vi "main_ctrl.vi"(8 "error in":errorcluster) -> (0 "error out":errorcluster caption="Error")   [LabVIEW 2013]
uses:
  <vilib>/Rock Robotics/WPI/DriverStation/WPI_DriverStationRobotMode2.ctl
  typedefs/fg_typedef.ctl
  typedefs/subStates.ctl
  typedefs/Loop Datatypes/Loop 1 Datatype.ctl
  typedefs/vision enable.ctl
  typedefs/singleUseSubstate.ctl
  <vilib>/Rock Robotics/WPI/Solenoid/WPI_SolenoidValue.ctl
  <vilib>/Rock Robotics/WPI/Compressor/WPI_CompressorGetSetRefNum.vi
  <vilib>/Rock Robotics/WPI/RobotDrive/WPI_RobotDriveGetSetRefNum.vi
  <vilib>/Rock Robotics/WPI/RobotDrive/WPI_RobotDriveArcadeDrive_Standard(NoSaturation).vi
  <vilib>/Rock Robotics/WPI/Solenoid/WPI_SolenoidSetEnum.vi
  typedefs/vision data.ctl
panel:
  out "Robot Mode":T1
  out "Vision SPI":u32
  out "Vision IPS":dbl
  out "Main IPS":dbl
  out "Main SPI":u32
  # "MAIN CONTROL"
  # "holds robot control code - dual parallel state machine"
  # "SPI: milliseconds per iteration\nIPS: iterations per second"
  # "need to incorporate cancel commands"
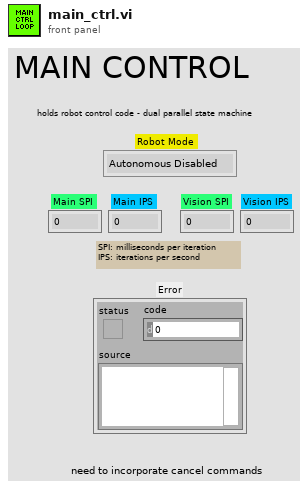
[diagram p1: front panel]
types:
  T1 = typedef "WPI_DriverStationRobotMode2.ctl" = enum16{"Autonomous Disabled", "Autonomous Enabled", "Teleop Disabled", "Teleop Enabled", "Timeout", "Finish", "Test Disabled", "Test Enabled"}
  T2 = typedef "vision data.ctl" = cluster{"x":dbl, "y":dbl, "area":dbl, "width":dbl, "height":dbl, "Hot Goal Present?":bool, "distance":dbl}
  T3 = typedef "vision enable.ctl" = enum16{"Enable", "Disable", "Stop"}
  T4 = typedef "fg_typedef.ctl" = enum16{"Get", "Set"}
  T5 = typedef "WPI_CameraDevRef.ctl" = cluster{"Camera Address":string, "CameraStatus":errorcluster, "Acquire Image Notifier":refnum<notifier>}
  T6 = typedef "IMAQ Image.ctl" = refnum<image>
  T7 = cluster{"Vision mSPI":u32, "Main mSPI":u32, "Dash mSPI":u32}
  T8 = typedef "WPI_RobotDriveDevRef.ctl" = cluster{"DevStatus":errorcluster, "Motors[]":T9[], "Square Inputs":bool, "Max Output":dbl, "Isochronous":bool}
  T9 = typedef "WPI_MotorControlDeviceRef.ctl" = cluster{"DeviceStatus":errorcluster, "Type":enum16{"PWM", "CAN"}, "PWM":cluster{"Digital Module":T10, "PWM Channel":T11, "DeadBand":T12}, "CAN":cluster{"Device Number":u8, "Control Mode":T13, "Semaphore":T14, "Max Vout":dbl}, "Invert":bool, "TransformRef":T15, "InvTransformRef":T15}
  T10 = typedef "FPGA_TypedefDigitalModule.ctl" = enum16{"Digital Module 1", "Digital Module 2"}
  T11 = typedef "FPGA_DIOPWMChannel.ctl" = enum8{"PWM 1", "PWM 2", "PWM 3", "PWM 4", "PWM 5", "PWM 6", "PWM 7", "PWM 8", "PWM 9", "PWM 10", "Invalid"}
  T12 = typedef "WPI_PWMDeadband.ctl" = cluster{"Name":string, "maxPositivePwm":i32, "minPositivePwm":i32, "centerPwm":i32, "maxNegativePwm":i32, "minNegativePwm":i32, "angularRange":u16}
  T13 = typedef "WPI_CANJaguar_ControlMode.ctl" = enum8{"Percent VBus", "Current", "Speed", "Position", "Voltage"}
  T14 = typedef "Semaphore RefNum" = refnum<k1>
  T15 = typedef "WPI_PWMTransform_ConPane.ctl" = refnum<vi>
  T16 = typedef "WPI_DigitalInputDevRef.ctl" = cluster{"DevStatus":errorcluster, "DIO Channel":T17, "Digital Module":T10}
  T17 = typedef "FPGA_DIOChannel.ctl" = enum8{"DIO 1", "DIO 2", "DIO 3", "DIO 4", "DIO 5", "DIO 6", "DIO 7", "DIO 8", "DIO 9", "DIO 10", "DIO 11", "DIO 12", "DIO 13", "DIO 14", "Invalid"}
  T18 = typedef "WPI_SolenoidDevRef.ctl" = cluster{"DevStatus":errorcluster, "Solenoid Module":T19, "Forward Solenoid Channel":T20, "Reverse Solenoid Channel":T20}
  T19 = typedef "FPGA_TypedefSolenoidModule.ctl" = enum16{"Solenoid Module 1", "Solenoid Module 2"}
  T20 = typedef "WPI_SolenoidChannel.ctl" = enum8{"Solenoid 1", "Solenoid 2", "Solenoid 3", "Solenoid 4", "Solenoid 5", "Solenoid 6", "Solenoid 7", "Solenoid 8", "Invalid"}
  T21 = typedef "WPI_CompressorDevRef.ctl" = cluster{"DevStatus":errorcluster, "DigitalInputDevRef":T16, "RelayDevRef":T22}
  T22 = typedef "WPI_RelayDevRef.ctl" = cluster{"DevStatus":errorcluster, "Relay Channel":T23, "Digital Module":T10, "Relay Direction":T24}
  T23 = typedef "FPGA_DIORelayChannel.ctl" = enum8{"Relay 1", "Relay 2", "Relay 3", "Relay 4", "Relay 5", "Relay 6", "Relay 7", "Relay 8", "Invalid"}
  T24 = typedef "WPI_RelayDirection.ctl" = enum16{"Both directions", "Forward only", "Reverse only"}
  T25 = typedef "Loop 1 Datatype.ctl" = cluster{"State":T26, "Waiting Loop":i32, "State to Wait For":i32, "Loop ID":i32, "Exit Value":i32}
  T26 = typedef "subStates.ctl" = enum16{"null", "wait", "driver control", "auto", "manual override", "hold position", "rotate", "pickup", "pass", "load", "goto shoot", "shoot", "cancel", "end"}
  T27 = typedef "WPI_SolenoidValue.ctl" = enum16{"Off", "On", "Forward", "Reverse"}
  T28 = typedef "singleUseSubstate.ctl" = enum16{"null", "wait", "shift high", "shift low", "extend shooter", "retract shooter", "close latch", "open latch"}
  T29 = typedef "WPI_DriverStationDerivedRobotMode.ctl" = enum16{"Init", "Execute", "Stop"}
  T30 = typedef "Loop 2 Datatype.ctl" = cluster{"State":T26, "Waiting Loop":i32, "State to Wait For":i32, "Loop ID":i32, "Exit Value":i32, "Joystick Y":dbl, "Tune Speed":dbl}
  T31 = typedef "Loop 3 Datatype.ctl" = cluster{"State":T26, "Waiting Loop":i32, "State to Wait For":i32, "Loop ID":i32, "Exit Value":i32, "Joystick Y":dbl, "Joystick Z":dbl}
  T32 = typedef "Loop 0 Datatype.ctl" = cluster{"State":T26, "Waiting Loop":i32, "State to Wait For":i32, "Loop ID":i32, "Exit Value":i32, "X Axis":dbl, "Y Axis":dbl, "Z Axis":dbl}
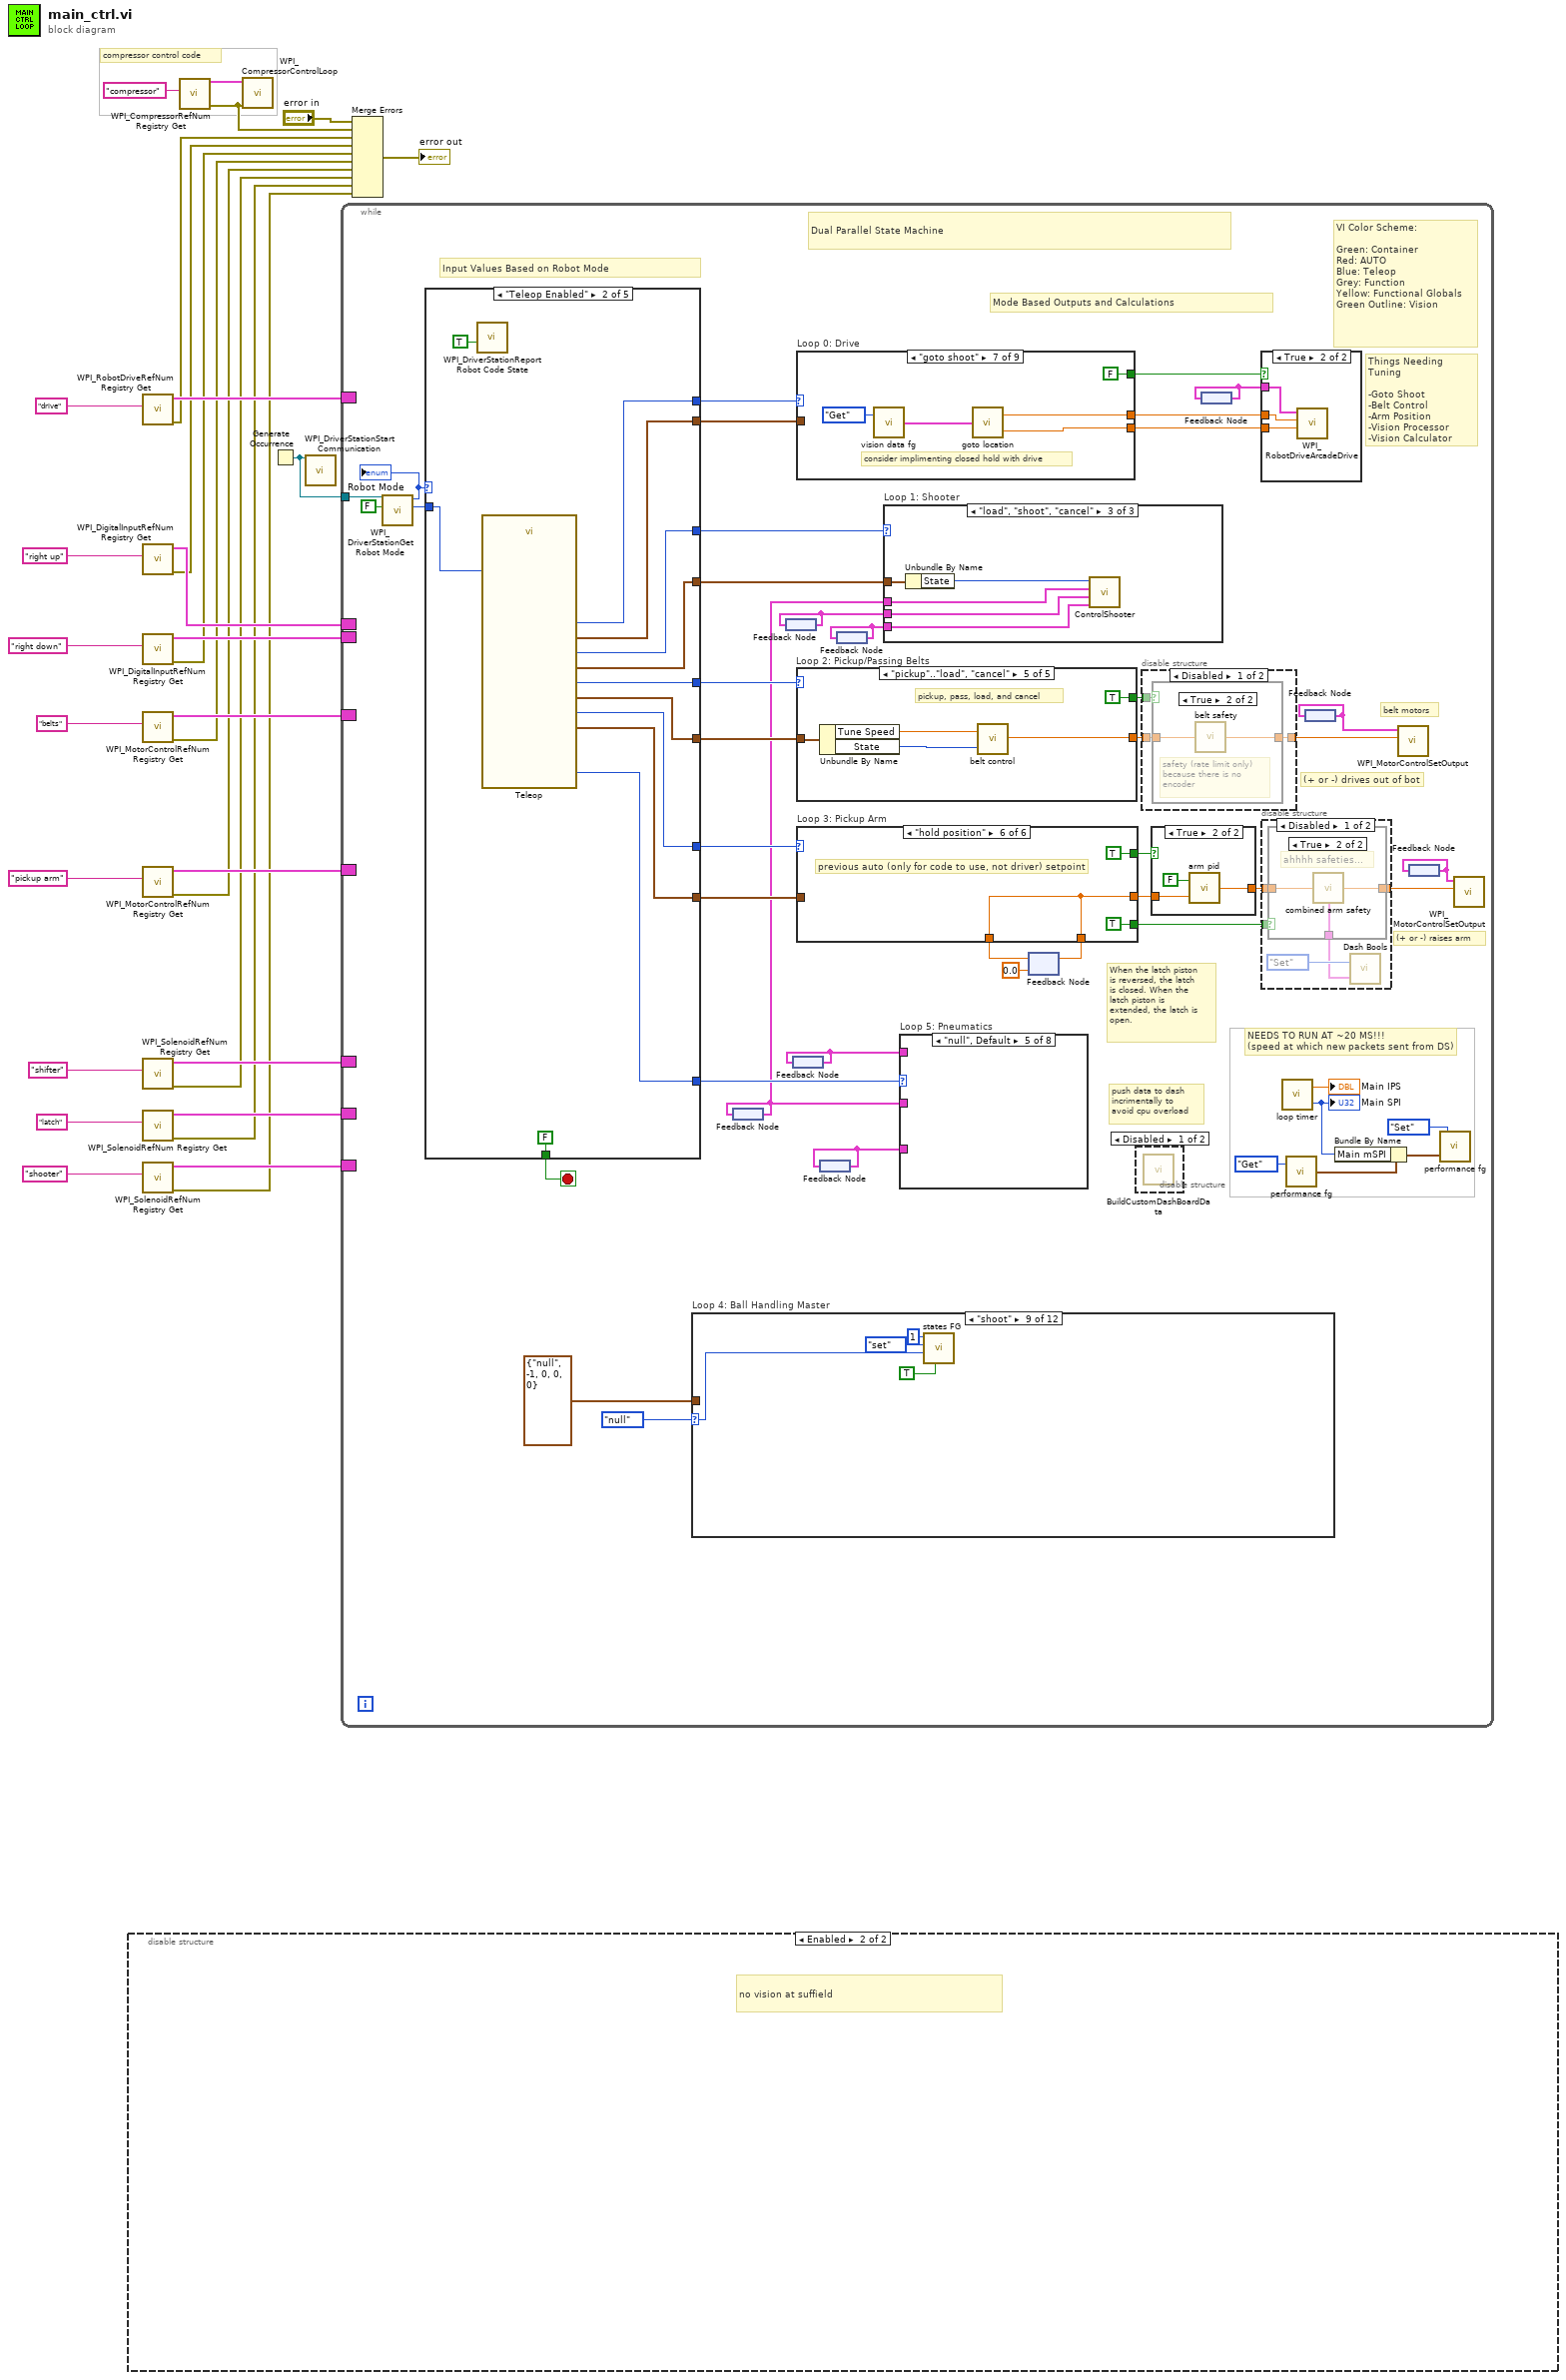
[diagram p0: block diagram]
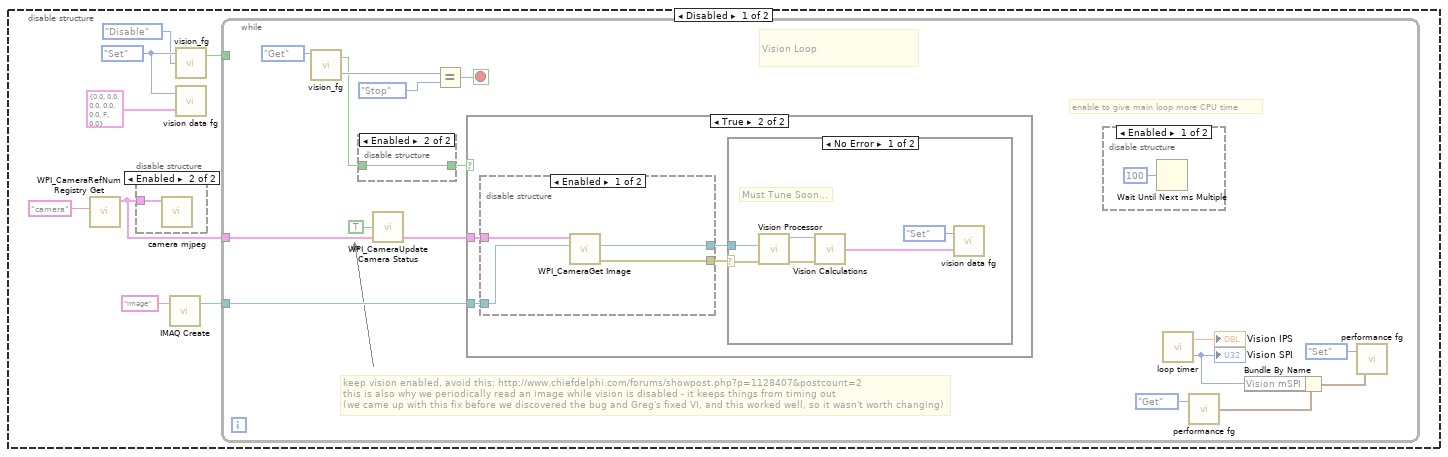
[diagram p2: hidden frame]
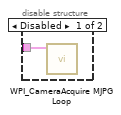
[diagram p3: hidden frame]
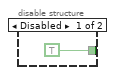
[diagram p4: hidden frame]
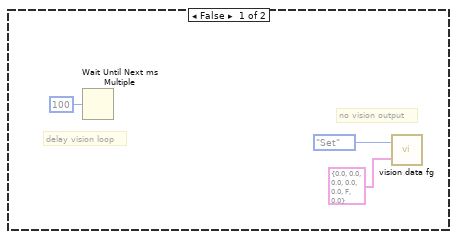
[diagram p6: hidden frame]
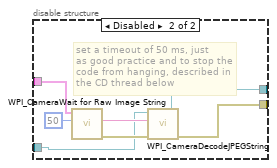
[diagram p8: hidden frame]
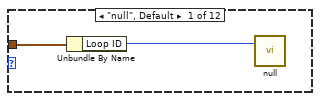
[diagram p9: hidden frame]
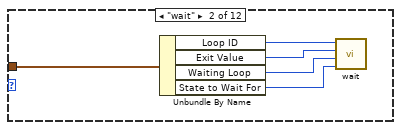
[diagram p10: hidden frame]
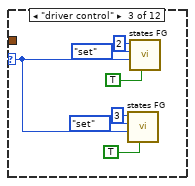
[diagram p11: hidden frame]
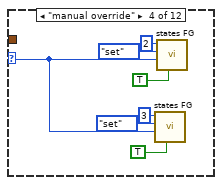
[diagram p12: hidden frame]
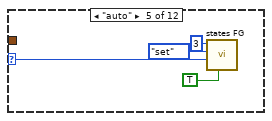
[diagram p13: hidden frame]
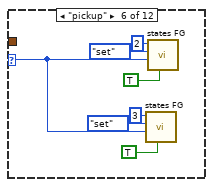
[diagram p14: hidden frame]
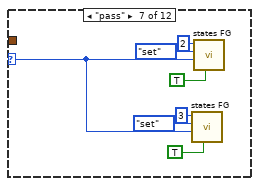
[diagram p15: hidden frame]
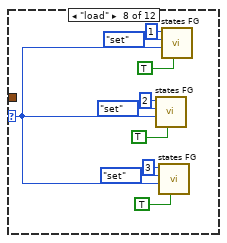
[diagram p16: hidden frame]
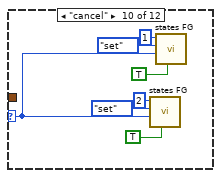
[diagram p17: hidden frame]
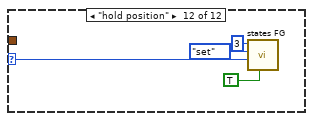
[diagram p19: hidden frame]
diagram:
  # "compressor control code"
  n1 = disable-structure shown="Enabled" {
    frame Disabled {
      w36 = fg_typedef."Set" ("Enum")
      n2 = call <vilib>:"WPI_CameraRefNum Registry Get.vi"("refnum name"="camera") -> ("CameraDevRef"=w33:T5)  [unwired: 9 in, 1 out]
      n3 = disable-structure shown="Enabled" {
        disable-tunnel: w33 -> [w39 w40]
        frame Disabled {
          n4 = call <vilib>:"WPI_CameraAcquire MJPG Loop.vi"("CameraDevRef"=w39) -> ()  [unwired: 11 in]
        }
        frame Enabled {
          n5 = call "camera mjpeg.vi"("CameraDevRef"=w40) -> ()  [unwired: 11 in]
        }
      }
      n6 = call "IMAQ Create"("Image Name"="image") -> ("New Image"=w38:T6)  [unwired: 4 in, 1 out]
      n7 = call "vision_fg.vi"("Action"=vision_enable."Disable", "Menu"=w36) -> ("Enabled?"=w37:bool)  [unwired: 1 in, 1 out]
      n8 = call "vision data fg.vi"("Input"=T2 {"x"=0.0, "y"=0.0, "area"=0.0, "width"=0.0, "height"=0.0, "Hot Goal Present?"=FALSE, "distance"=0.0} ("Cluster"), "Menu"=w36) -> ()  [unwired: 1 out]
      n9 = while {
        tunnel: w38 -> [w55]
        tunnel: w33 -> [w54]
        tunnel: w37 -> [_]
        stop <- w56 stop-if-true
        # "keep vision enabled, avoid this: http://www.chiefdelphi.com/forums/showpost.php?p=1128407&postcount=2\nthis is also why we periodically read an image while vision is disabled - it keeps things from timing out\n(we came up with this fix before we discovered the bug and Greg's fixed VI, and this worked well, so it wasn't worth changing)"
        # "enable to give main loop more CPU time"
        # "Vision Loop"
        n10 = call "vision_fg.vi"("Menu"=fg_typedef."Get" ("Enum")) -> ("State Out"=w50:T3, "Enabled?"=w41:bool)  [unwired: 2 in]
        n11 = disable-structure shown="Enabled" {
          disable-tunnel: [TRUE w58] -> w42
          disable-tunnel: w41 -> [_ w58]
          frame Disabled {
          }
          frame Enabled {
          }
        }
        n12 = call <vilib>:"WPI_CameraUpdate Camera Status.vi"("CameraDevRef In"=w54, "Enable Vision"=TRUE) -> ("CameraDevRef Out"=w53:T5)  [unwired: 3 in]
        n13 = Equal?(x=w50, y=vision_enable."Stop") -> (x = y?=w56:bool)
        n14 = case shown="True" w42 {
          tunnel: w55 -> [_ w66]
          tunnel: w53 -> [_ w65]
          frame False {
            # "no vision output"
            # "delay vision loop"
            n15 = Wait Until Next ms Multiple(millisecond multiple=u32 100) -> ()  [unwired: 1 out]
            n16 = call "vision data fg.vi"("Input"=T2 {"x"=0.0, "y"=0.0, "area"=0.0, "width"=0.0, "height"=0.0, "Hot Goal Present?"=FALSE, "distance"=0.0} ("Cluster"), "Menu"=fg_typedef."Set" ("Enum")) -> ()  [unwired: 1 out]
          }
          frame True {
            n17 = disable-structure shown="Enabled" {
              disable-tunnel: w66 -> [w75 w79]
              disable-tunnel: w65 -> [w76 w81]
              disable-tunnel: [w74 w78] -> w64
              disable-tunnel: [w73 w77] -> w63
              frame Enabled {
                n18 = call <vilib>:"WPI_CameraGet Image.vi"("Image"=w75, "CameraDevRef"=w76) -> ("error out"=w73:errorcluster, "Image Out"=w74:T6)  [unwired: 7 in, 1 out]
              }
              frame Disabled {
                # "set a timeout of 50 ms, just\nas good practice and to stop the \ncode from hanging, described in \nthe CD thread below"
                n19 = call <vilib>:"WPI_CameraWait for Raw Image String.vi"("Timeout in ms (-1)"=50, "CameraDevRef"=w81) -> ("error out"=w83:errorcluster, "String"=w82:string)  [unwired: 3 in, 5 out]
                n20 = call <vilib>:"WPI_CameraDecodeJPEGString.vi"("error in"=w83, "Compressed Image"=w82, "Image In"=w79) -> ("error out"=w77:errorcluster, "Image Out"=w78:T6)  [unwired: 3 out]
              }
            }
            n21 = case shown="No Error" w63 {
              selector: w63 -> [w71 _]
              tunnel: w64 -> [w70 _]
              frame No Error {
                # "Must Tune Soon..."
                n22 = call "Vision Processor.vi"("error in"=w71, "Image In"=w70) -> ("error out"=w68:errorcluster, "Image Out"=w69:T6)  [unwired: 5 in]
                n23 = call "Vision Calculations.vi"("Image In"=w69, "error in"=w68) -> ("Vision Data"=w67:T2)  [unwired: 3 in]
                n24 = call "vision data fg.vi"("Input"=w67, "Menu"=fg_typedef."Set" ("Enum")) -> ()  [unwired: 1 out]
              }
              frame Error {
              }
            }
          }
        }
        n25 = disable-structure shown="Enabled" {
          frame Enabled {
            n26 = Wait Until Next ms Multiple(millisecond multiple=u32 100) -> ()  [unwired: 1 out]
          }
          frame Disabled {
          }
        }
        n27 = call "loop timer.vi"() -> ("IPS"=→"Vision IPS":dbl, "SPI"=w48:u32)  [unwired: 1 in]
        "Vision SPI" <- w48
        n28 = call "performance fg.vi"("Menu"=fg_typedef."Get") -> ("Output"=w46:T7)  [unwired: 1 in]
        n29 = Bundle By Name(cluster=w46, "Vision mSPI"=w48) -> (w45:T7)
        n30 = call "performance fg.vi"("Input"=w45, "Menu"=fg_typedef."Set") -> ()  [unwired: 1 out]
      }
    }
    frame Enabled {
      # "no vision at suffield"
    }
  }
  n31 = call <vilib>:"WPI_RobotDriveRefNum Registry Get.vi"("refnum name"="drive") -> ("error out"=w10:errorcluster, "RobotDriveDevRef"=w27:T8)  [unwired: 9 in]
  n32 = call <vilib>:"WPI_DigitalInputRefNum Registry Get.vi"("refnum name"="right up") -> ("error out"=w9:errorcluster, "DigitalInputDevRef"=w12:T16)  [unwired: 9 in]
  n33 = call <vilib>:"WPI_DigitalInputRefNum Registry Get.vi"("refnum name"="right down") -> ("error out"=w8:errorcluster, "DigitalInputDevRef"=w11:T16)  [unwired: 9 in]
  n34 = call <vilib>:"WPI_MotorControlRefNum Registry Get.vi"("refnum name"="belts") -> ("error out"=w7:errorcluster, "MotorControlDevRef"=w18:T9)  [unwired: 9 in]
  n35 = call <vilib>:"WPI_MotorControlRefNum Registry Get.vi"("refnum name"="pickup arm") -> ("error out"=w6:errorcluster, "MotorControlDevRef"=w15:T9)  [unwired: 9 in]
  n36 = call <vilib>:"WPI_SolenoidRefNum Registry Get.vi"("refnum name"="shifter") -> ("error out"=w5:errorcluster, "SolenoidDevRef"=w25:T18)  [unwired: 9 in]
  n37 = call <vilib>:"WPI_SolenoidRefNum Registry Get.vi"("refnum name"="latch") -> ("error out"=w4:errorcluster, "SolenoidDevRef"=w19:T18)  [unwired: 9 in]
  n38 = call <vilib>:"WPI_SolenoidRefNum Registry Get.vi"("refnum name"="shooter") -> ("error out"=w3:errorcluster, "SolenoidDevRef"=w21:T18)  [unwired: 9 in]
  n39 = call <vilib>:"WPI_CompressorRefNum Registry Get.vi"("refnum name"="compressor") -> ("error out"=w1:errorcluster, "CompressorDevRef"=w26:T21)  [unwired: 9 in]
  n40 = call <vilib>:"WPI_CompressorControlLoop.vi"("error in (no error)"=w1, "CompressorDevRef"=w26) -> ()  [unwired: 10 in]
  n41 = Generate Occurrence() -> (w23:refnum<k4>)
  n42 = call <vilib>:"WPI_DriverStationStart Communication.vi"("occurrence"=w23) -> ()  [unwired: 11 in]
  n43 = while {
    tunnel: w23 -> [w105]
    border: w27 -> [_]
    border: w25 -> [_]
    border: w21 -> [_]
    border: w19 -> [_]
    border: w18 -> [_]
    border: w15 -> [_]
    border: w12 -> [_]
    border: w11 -> [_]
    stop <- w124 stop-if-true
    # "When the latch piston\nis reversed, the latch\nis closed. When the\nlatch piston is\nextended, the latch is\nopen."
    # "push data to dash \nincrimentally to\navoid cpu overload"
    # "Things Needing Tuning\n\n-Goto Shoot\n-Belt Control\n-Arm Position\n-Vision Processor\n-Vision Calculator"
    # "(+ or -) raises arm"
    # "(+ or -) drives out of bot"
    # "belt motors"
    # "VI Color Scheme:\n\nGreen: Container\nRed: AUTO\nBlue: Teleop\nGrey: Function\nYellow: Functional Globals\nGreen Outline: Vision"
    # "Input Values Based on Robot Mode"
    # "Mode Based Outputs and Calculations"
    # "NEEDS TO RUN AT ~20 MS!!!\n(speed at which new packets sent from DS)"
    # "Dual Parallel State Machine"
    n44 = call <vilib>:"WPI_DriverStationGet Robot Mode.vi"("Finish"=FALSE, "DS Occurrence"=w105) -> ("Call Context"=w104:T29, "Robot Mode"=w103:T1)  [unwired: 8 out]
    "Robot Mode" <- w103
    n45 = case shown="\"Teleop Enabled\"" w103 {
      tunnel: [w378 w393 w395 w401 w407] -> w107
      tunnel: w104 -> [w371 w389 _ _ _]
      tunnel: [w376 w392 w395 w401 w407] -> w126
      tunnel: [w372 w390 singleUseSubstate."null" ("SubState 5") singleUseSubstate."null" ("SubState 5") singleUseSubstate."null" ("SubState 5")] -> w125
      tunnel: [FALSE FALSE FALSE FALSE TRUE] -> w124
      tunnel: [w380 w388 w395 w401 w407] -> w117
      tunnel: [w379 w387 _ _ _] -> w118
      tunnel: [w377 w386 _ _ _] -> w116
      tunnel: [w375 w385 _ _ _] -> w115
      tunnel: [w373 w384 _ _ _] -> w113
      tunnel: [w374 w383 w395 w401 w407] -> w112
      frame "Autonomous Enabled" {
        n46 = call <vilib>:"WPI_DriverStationReport Robot Code State.vi"("Autonomous"=TRUE) -> ()  [unwired: 10 in, 1 out]
        n47 = call "Autonomous.vi"("Call Context"=w371) -> ("SubState 2"=w376:T26, "Loop 2 Data"=w375:T30, "SubState 1"=w378:T26, "Loop 1 Data"=w377:T25, "Loop 3 Data"=w373:T31, "SubState 0"=w380:T26, "SubState 3"=w374:T26, "Loop 0 Data"=w379:T32, "SubState 5"=w372:T28)  [unwired: 2 out]
      }
      frame "Teleop Enabled" {
        n48 = call <vilib>:"WPI_DriverStationReport Robot Code State.vi"("TeleOp"=TRUE) -> ()  [unwired: 10 in, 1 out]
        n49 = call "Teleop.vi"("Call Context"=w389) -> ("SubState 3"=w383:T26, "SubState 5"=w390:T28, "Loop 3 Data"=w384:T31, "SubState 0"=w388:T26, "Loop 1 Data"=w386:T25, "Loop 0 Data"=w387:T32, "SubState 1"=w393:T26, "Loop 2 Data"=w385:T30, "SubState 2"=w392:T26)  [unwired: 8 in, 2 out]
      }
      frame "Autonomous Disabled", "Teleop Disabled", "Timeout" {
        w395 = subStates."null" ("SubState 0")
        # "set all loops to null"
        # "make sure to disable vision\nwe don't need it here"
        # "robot disabled, timeout"
        n50 = call <vilib>:"WPI_DriverStationReport Robot Code State.vi"("Disabled"=TRUE) -> ()  [unwired: 10 in, 1 out]
        n51 = call "vision_fg.vi"("Action"=vision_enable."Disable", "Menu"=fg_typedef."Set") -> ()  [unwired: 1 in, 2 out]
      }
      frame "Test Disabled", "Test Enabled" {
        w401 = subStates."null" ("SubState 0")
        # "set all loops to null"
        # "make sure to disable vision\nwe don't need it here"
        # "test, unused"
        n52 = call <vilib>:"WPI_DriverStationReport Robot Code State.vi"("Test"=TRUE) -> ()  [unwired: 10 in, 1 out]
        n53 = call "vision_fg.vi"("Action"=vision_enable."Disable", "Menu"=fg_typedef."Set") -> ()  [unwired: 1 in, 2 out]
      }
      frame "Finish" {
        w407 = subStates."end"  # Stop All Loops
        # "stop the while loop"
        # "stop DS comms"
        # "stop vision loop"
        n54 = call <vilib>:"WPI_DriverStationStop Communication.vi"("StopCommunication"=TRUE) -> ()  [unwired: 10 in, 1 out]
        n55 = call "vision_fg.vi"("Action"=vision_enable."Stop", "Menu"=fg_typedef."Set") -> ()  [unwired: 1 in, 2 out]
      }
    }
    n56 = case "Loop 4: Ball Handling Master" shown="\"shoot\"" subStates."null" ("Stop All Loops") {
      selector: subStates."null" ("Stop All Loops") -> [_ _ w135 w142 w149 w153 w160 w167 w177 w181 _ w188]
      tunnel: T25 {"State"=enum."null", "Waiting Loop"=-1, "State to Wait For"=0, "Loop ID"=0, "Exit Value"=0} ("input cluster") -> [w129 w130 _ _ _ _ _ _ _ _ _ _]
      frame "null", Default {
        n57 = Unbundle By Name(w129) -> ("Loop ID"=w128:i32)
        n58 = call "null.vi"("This Loop ID"=w128) -> ()  [unwired: 2 in]
      }
      frame "wait" {
        n59 = Unbundle By Name(w130) -> ("Loop ID"=w134:i32, "Exit Value"=w133:i32, "Waiting Loop"=w132:i32, "State to Wait For"=w131:i32)
        n60 = call "wait.vi"("State to wait for"=w131, "Waiting Loop ID"=w132, "time (ms)"=w133, "Current Loop ID"=w134) -> ()  [unwired: 1 out]
      }
      frame "driver control" {
        n61 = call "states FG.vi"("exit in"=TRUE, "subState in"=w135, "menu (get)"=enum16{"set", "get"}."set", "Loop ID"=3) -> ()  [unwired: 4 in, 4 out]
        n62 = call "states FG.vi"("exit in"=TRUE, "subState in"=w135, "menu (get)"=enum16{"set", "get"}."set", "Loop ID"=2) -> ()  [unwired: 4 in, 4 out]
      }
      frame "manual override" {
        n63 = call "states FG.vi"("exit in"=TRUE, "subState in"=w142, "menu (get)"=enum16{"set", "get"}."set", "Loop ID"=3) -> ()  [unwired: 4 in, 4 out]
        n64 = call "states FG.vi"("exit in"=TRUE, "subState in"=w142, "menu (get)"=enum16{"set", "get"}."set", "Loop ID"=2) -> ()  [unwired: 4 in, 4 out]
      }
      frame "auto" {
        n65 = call "states FG.vi"("exit in"=TRUE, "subState in"=w149, "menu (get)"=enum16{"set", "get"}."set", "Loop ID"=3) -> ()  [unwired: 4 in, 4 out]
      }
      frame "pickup" {
        n66 = call "states FG.vi"("exit in"=TRUE, "subState in"=w153, "menu (get)"=enum16{"set", "get"}."set", "Loop ID"=3) -> ()  [unwired: 4 in, 4 out]
        n67 = call "states FG.vi"("exit in"=TRUE, "subState in"=w153, "menu (get)"=enum16{"set", "get"}."set", "Loop ID"=2) -> ()  [unwired: 4 in, 4 out]
      }
      frame "pass" {
        n68 = call "states FG.vi"("exit in"=TRUE, "subState in"=w160, "menu (get)"=enum16{"set", "get"}."set", "Loop ID"=3) -> ()  [unwired: 4 in, 4 out]
        n69 = call "states FG.vi"("exit in"=TRUE, "subState in"=w160, "menu (get)"=enum16{"set", "get"}."set", "Loop ID"=2) -> ()  [unwired: 4 in, 4 out]
      }
      frame "load" {
        n70 = call "states FG.vi"("exit in"=TRUE, "subState in"=w167, "menu (get)"=enum16{"set", "get"}."set", "Loop ID"=2) -> ()  [unwired: 4 in, 4 out]
        n71 = call "states FG.vi"("exit in"=TRUE, "subState in"=w167, "menu (get)"=enum16{"set", "get"}."set", "Loop ID"=3) -> ()  [unwired: 4 in, 4 out]
        n72 = call "states FG.vi"("exit in"=TRUE, "subState in"=w167, "menu (get)"=enum16{"set", "get"}."set", "Loop ID"=1) -> ()  [unwired: 4 in, 4 out]
      }
      frame "shoot" {
        n73 = call "states FG.vi"("exit in"=TRUE, "subState in"=w177, "menu (get)"=enum16{"set", "get"}."set", "Loop ID"=1) -> ()  [unwired: 4 in, 4 out]
      }
      frame "cancel" {
        n74 = call "states FG.vi"("exit in"=TRUE, "subState in"=w181, "menu (get)"=enum16{"set", "get"}."set", "Loop ID"=2) -> ()  [unwired: 4 in, 4 out]
        n75 = call "states FG.vi"("exit in"=TRUE, "subState in"=w181, "menu (get)"=enum16{"set", "get"}."set", "Loop ID"=1) -> ()  [unwired: 4 in, 4 out]
      }
      frame "end" {
      }
      frame "hold position" {
        n76 = call "states FG.vi"("exit in"=TRUE, "subState in"=w188, "menu (get)"=enum16{"set", "get"}."set", "Loop ID"=3) -> ()  [unwired: 4 in, 4 out]
      }
    }
    n77 = feedback #1() -> (w86:T18)
    n78 = feedback-in #1(w86) -> ()
    n79 = feedback #2() -> (w88:T16)
    n80 = feedback-in #2(w88) -> ()
    n81 = feedback #3() -> (w114:T18)
    n82 = feedback-in #3(w114) -> ()
    n83 = case "Loop 0: Drive" shown="\"goto shoot\"" w117 {
      tunnel: w118 -> [w222 w226 w238 w245 w262 w269 _ _ w285]
      tunnel: [w220 w224 w236 w247 w259 w271 w274 w279 w281] -> w110
      tunnel: [w220 w224 w235 w246 w258 w270 w273 w279 w280] -> w109
      tunnel: [FALSE FALSE TRUE FALSE FALSE FALSE FALSE FALSE FALSE] -> w111
      frame "null", Default {
        w220 = 0.0 ("X Axis")
        n84 = Unbundle By Name(w222) -> ("Loop ID"=w223:i32)
        n85 = call "null.vi"("This Loop ID"=w223) -> ()  [unwired: 2 in]
      }
      frame "wait" {
        w224 = 0.0 ("X Axis")
        n86 = Unbundle By Name(w226) -> ("Loop ID"=w230:i32, "Exit Value"=w229:i32, "Waiting Loop"=w228:i32, "State to Wait For"=w227:i32)
        n87 = call "wait.vi"("State to wait for"=w227, "Waiting Loop ID"=w228, "time (ms)"=w229, "Current Loop ID"=w230) -> ()  [unwired: 1 out]
      }
      frame "driver control" {
        # "filter joysticks"
        n88 = Unbundle By Name(w238) -> ("X Axis"=w231:dbl, "Y Axis"=w234:dbl)
        n89 = call "Joystick Error Filter.vi"("Axis"=w231) -> ("Filtered Axis"=w232:dbl)
        n90 = call "Joystick Error Filter.vi"("Axis"=w234) -> ("Filtered Axis"=w233:dbl)
        n91 = disable-structure shown="Enabled" {
          disable-tunnel: w232 -> [w242 w244]
          disable-tunnel: w233 -> [w241 w243]
          disable-tunnel: [w240 w244] -> w236
          disable-tunnel: [w239 w243] -> w235
          frame Disabled {
            n92 = call "calc arcade drive pwm.vi"("Y axis value"=w241, "X axis value"=w242) -> ("Right Speed"=w239:dbl, "Left Speed"=w240:dbl)  [unwired: 1 in, 1 out]
          }
          frame Enabled {
          }
        }
      }
      frame "auto" {
        n93 = disable-structure shown="Enabled" {
          disable-tunnel: [w256 _] -> w247
          disable-tunnel: [w255 _] -> w246
          disable-tunnel: w245 -> [w251 _]
          frame Disabled {
            n94 = Unbundle By Name(w251) -> ("Z Axis"=w249:dbl)
            n95 = call "Vision Tracking X.vi"("Tweak"=w249) -> ("right speed"=w250:dbl, "left speed"=w253:dbl)
            n96 = call "closed drive.vi"("Acrade Drive?"=FALSE, "Y axis value (Left)"=w253, "X axis value (Right)"=w250, "Threshold (.4)"=0.0 ("Threshold")) -> ("right"=w255:dbl, "left"=w256:dbl)
          }
          frame Enabled {
            # "rotates toward target"
            # "not in use this year"
          }
        }
      }
      frame "hold position" {
        n97 = Unbundle By Name(w262) -> ("X Axis"=w261:dbl, "Y Axis"=w260:dbl)
        n98 = call "closed drive.vi"("Acrade Drive?"=TRUE, "Y axis value (Left)"=w260, "X axis value (Right)"=w261) -> ("right"=w258:dbl, "left"=w259:dbl)  [unwired: 1 in]
      }
      frame "rotate" {
        # "use these to carry actual information because this is\nfor autonomous only so there will not be joystick input"
        n99 = Unbundle By Name(w269) -> ("X Axis"=w268:dbl, "Y Axis"=w267:dbl)
        n100 = call "rotate.vi"("Angle"=w268, "Rate"=w267) -> ("finished?"=w264:bool, "left speed"=w271:dbl, "right speed"=w270:dbl)
        n101 = call "states FG.vi"("exit in"=w264, "menu (get)"=enum16{"set", "get"}."set", "Loop ID"=0) -> ()  [unwired: 5 in, 4 out]
      }
      frame "goto shoot" {
        # "consider implimenting closed hold with drive"
        n102 = call "vision data fg.vi"("Menu"=fg_typedef."Get") -> ("Output"=w275:T2)  [unwired: 1 in]
        n103 = call "goto location.vi"("Image Data"=w275) -> ("left speed"=w274:dbl, "right speed"=w273:dbl)
      }
      frame "end" {
        w279 = 0.0 ("X Axis")
      }
      frame "manual override" {
        n104 = Unbundle By Name(w285) -> ("X Axis"=w284:dbl, "Y Axis"=w283:dbl)
        n105 = expression code="x/2"(w284) -> (w281:dbl)
        n106 = expression code="x/2"(w283) -> (w280:dbl)
      }
    }
    n107 = case "Loop 2: Pickup/Passing Belts" shown="\"pickup\"..\"load\", \"cancel\"" w126 {
      tunnel: w115 -> [w337 w340 w348 w352 w357]
      tunnel: [0.0 ("output") 0.0 ("output") w346 w350 w354] -> w94
      tunnel: [FALSE FALSE TRUE FALSE TRUE] -> w95
      frame "null", Default {
        n108 = Unbundle By Name(w337) -> ("Loop ID"=w336:i32)
        n109 = call "null.vi"("This Loop ID"=w336) -> ()  [unwired: 2 in]
      }
      frame "wait" {
        n110 = Unbundle By Name(w340) -> ("Loop ID"=w344:i32, "Exit Value"=w343:i32, "Waiting Loop"=w342:i32, "State to Wait For"=w341:i32)
        n111 = call "wait.vi"("State to wait for"=w341, "Waiting Loop ID"=w342, "time (ms)"=w343, "Current Loop ID"=w344) -> ()  [unwired: 1 out]
      }
      frame "driver control" {
        n112 = Unbundle By Name(w348) -> ("Joystick Y"=w345:dbl)
        n113 = call "Joystick Error Filter.vi"("Axis"=w345) -> ("Filtered Axis"=w346:dbl)
      }
      frame "manual override" {
        n114 = Unbundle By Name(w352) -> ("Joystick Y"=w351:dbl)
        n115 = expression code="x/2"(w351) -> (w350:dbl)
      }
      frame "pickup".."load", "cancel" {
        # "pickup, pass, load, and cancel"
        n116 = Unbundle By Name(w357) -> ("Tune Speed"=w356:dbl, "State"=w355:T26)
        n117 = call "belt control.vi"("State"=w355, "Joystick Z"=w356) -> ("output"=w354:dbl)
      }
    }
    n118 = feedback #4() -> (w89:T18)
    n119 = feedback-in #4(w89) -> ()
    n120 = feedback #5() -> (w87:T16)
    n121 = feedback-in #5(w87) -> ()
    n122 = case "Loop 1: Shooter" shown="\"load\", \"shoot\", \"cancel\"" w107 {
      tunnel: w116 -> [w358 w360 w369]
      tunnel: w86 -> [_ _ w367]
      tunnel: w88 -> [_ _ w366]
      tunnel: w87 -> [_ _ w365]
      frame "null", Default {
        n123 = Unbundle By Name(w358) -> ("Loop ID"=w359:i32)
        n124 = call "null.vi"("This Loop ID"=w359) -> ()  [unwired: 2 in]
      }
      frame "wait" {
        n125 = Unbundle By Name(w360) -> ("Loop ID"=w364:i32, "Exit Value"=w363:i32, "Waiting Loop"=w362:i32, "State to Wait For"=w361:i32)
        n126 = call "wait.vi"("State to wait for"=w361, "Waiting Loop ID"=w362, "time (ms)"=w363, "Current Loop ID"=w364) -> ()  [unwired: 1 out]
      }
      frame "load", "shoot", "cancel" {
        n127 = Unbundle By Name(w369) -> ("State"=w368:T26)
        n128 = call "ControlShooter.vi"("right down"=w365, "right up"=w366, "latch"=w367, "State"=w368) -> ()  [unwired: 1 in]
      }
    }
    n129 = case "Loop 5: Pneumatics" shown="\"null\", Default" w125 {
      tunnel: w114 -> [_ _ _ _ _ _ w331 w332]
      tunnel: w86 -> [w322 w324 _ _ _ _ _ _]
      tunnel: w89 -> [_ _ w326 w328 _ _ _ _]
      frame "open latch" {
        n130 = call-poly <vilib>:"WPI_SolenoidSet.vi"("Value"=WPI_SolenoidValue."Forward", "SolenoidDevRef"=w322) -> ()  [unwired: 8 in, 2 out]
      }
      frame "close latch" {
        n131 = call-poly <vilib>:"WPI_SolenoidSet.vi"("Value"=WPI_SolenoidValue."Forward", "SolenoidDevRef"=w324) -> ()  [unwired: 8 in, 2 out]
      }
      frame "retract shooter" {
        n132 = call-poly <vilib>:"WPI_SolenoidSet.vi"("Value"=WPI_SolenoidValue."Reverse", "SolenoidDevRef"=w326) -> ()  [unwired: 8 in, 2 out]
      }
      frame "extend shooter" {
        n133 = call-poly <vilib>:"WPI_SolenoidSet.vi"("Value"=WPI_SolenoidValue."Forward", "SolenoidDevRef"=w328) -> ()  [unwired: 8 in, 2 out]
      }
      frame "null", Default {
      }
      frame "wait" {
      }
      frame "shift high" {
        n134 = call-poly <vilib>:"WPI_SolenoidSet.vi"("Value"=WPI_SolenoidValue."Forward", "SolenoidDevRef"=w331) -> ()  [unwired: 8 in, 2 out]
      }
      frame "shift low" {
        n135 = call-poly <vilib>:"WPI_SolenoidSet.vi"("Value"=WPI_SolenoidValue."Reverse", "SolenoidDevRef"=w332) -> ()  [unwired: 8 in, 2 out]
      }
    }
    n136 = feedback #6(0.0 ("setpoint")) -> (w91:dbl)
    n137 = case "Loop 3: Pickup Arm" shown="\"hold position\"" w112 {
      tunnel: w113 -> [w291 w296 w305 w312 w318 _]
      tunnel: [FALSE FALSE FALSE FALSE TRUE TRUE] -> w100
      tunnel: [0.0 ("output") 0.0 ("output") w302 w310 w313 w319] -> w99
      tunnel: [TRUE TRUE TRUE FALSE TRUE TRUE] -> w98
      tunnel: [w286 w292 w301 w307 w313 w319] -> w92
      tunnel: w91 -> [w286 w292 w301 w307 _ w319]
      frame "null", Default {
        n138 = Unbundle By Name(w291) -> ("Loop ID"=w290:i32)
        n139 = call "null.vi"("This Loop ID"=w290) -> ()  [unwired: 2 in]
      }
      frame "wait" {
        n140 = Unbundle By Name(w296) -> ("Loop ID"=w300:i32, "Exit Value"=w299:i32, "Waiting Loop"=w298:i32, "State to Wait For"=w297:i32)
        n141 = call "wait.vi"("State to wait for"=w297, "Waiting Loop ID"=w298, "time (ms)"=w299, "Current Loop ID"=w300) -> ()  [unwired: 1 out]
      }
      frame "driver control" {
        n142 = Unbundle By Name(w305) -> ("Joystick Y"=w303:dbl)
        n143 = call "Joystick Error Filter.vi"("Axis"=w303) -> ("Filtered Axis"=w302:dbl)
      }
      frame "manual override" {
        n144 = Unbundle By Name(w312) -> ("Joystick Y"=w311:dbl)
        n145 = expression code="x/2"(w311) -> (w310:dbl)
      }
      frame "auto", "pickup".."load" {
        # "pickup, pass, auto, and load"
        n146 = Unbundle By Name(w318) -> ("Joystick Z"=w316:dbl, "State"=w315:T26)
        n147 = call "arm control.vi"("State"=w315, "Z Axis (Tuning)"=w316) -> ("setpoint"=w313:dbl)
      }
      frame "hold position" {
        # "previous auto (only for code to use, not driver) setpoint"
      }
    }
    n148 = feedback-in #6(w92) -> ()
    n149 = disable-structure shown="Disabled" {
      frame Disabled {
        n150 = call "BuildCustomDashBoardData.vi"() -> ()  [unwired: 12 in]
      }
      frame Enabled {
      }
    }
    n151 = disable-structure shown="Disabled" {
      disable-tunnel: w95 -> [w209 _]
      disable-tunnel: w94 -> [w208 _]
      disable-tunnel: [w207 0.0 ("Output")] -> w93
      frame Disabled {
        n152 = case shown="True" w209 {
          tunnel: w208 -> [w210 w212]
          tunnel: [w210 w211] -> w207
          frame False {
            # "no safety"
          }
          frame True {
            # "safety (rate limit only)\nbecause there is no \nencoder"
            n153 = call "belt safety.vi"("Input"=w212) -> ("Safe Output"=w211:dbl)
          }
        }
      }
      frame Enabled {
      }
    }
    n154 = case shown="True" w100 {
      tunnel: w99 -> [w192 w195]
      tunnel: [w192 w193] -> w97
      frame False {
        # "open loop"
      }
      frame True {
        n155 = call "arm pid.vi"("Setpoint"=w195, "Autotune?"=FALSE) -> ("Output"=w193:dbl)
      }
    }
    n156 = feedback #7() -> (w108:T8)
    n157 = feedback-in #7(w108) -> ()
    n158 = case shown="True" w111 {
      tunnel: w110 -> [w215 w219]
      tunnel: w109 -> [w214 w218]
      tunnel: w108 -> [w216 w217]
      frame False {
        n159 = call <vilib>:"WPI_RobotDriveMotors.vi"("RightSpeed"=w214, "LeftSpeed"=w215, "RobotDriveDevRef"=w216) -> ()  [unwired: 6 in, 3 out]
      }
      frame True {
        n160 = call-poly <vilib>:"WPI_RobotDriveArcadeDrive.vi"("Y axis value"=w218, "X axis value"=w219, "RobotDriveDevRef"=w217) -> ()  [unwired: 6 in, 3 out]
      }
    }
    n161 = disable-structure shown="Disabled" {
      disable-tunnel: w98 -> [w200 _]
      disable-tunnel: w97 -> [w199 _]
      disable-tunnel: [w198 0.0 ("Output")] -> w96
      frame Disabled {
        n162 = case shown="True" w200 {
          tunnel: w199 -> [w202 w205]
          tunnel: [w202 w204] -> w198
          tunnel: [cluster{"Arm Safety":bool, "Arm Limit":bool} {"Arm Safety"=FALSE, "Arm Limit"=FALSE} ("Input") w203] -> w196
          frame False {
            # "no safety???"
          }
          frame True {
            # "ahhhh safeties..."
            n163 = call "combined arm safety.vi"("Input"=w205) -> ("Safe Output"=w204:dbl, "Safety"=w203:cluster{"Arm Safety":bool, "Arm Limit":bool})  [unwired: 13 in]
          }
        }
        n164 = call "Dash Bools.vi"("Input"=w196, "Menu"=fg_typedef."Set") -> ()  [unwired: 1 out]
      }
      frame Enabled {
      }
    }
    n165 = call "loop timer.vi"() -> ("IPS"=→"Main IPS":dbl, "SPI"=w123:u32)  [unwired: 1 in]
    "Main SPI" <- w123
    n166 = call "performance fg.vi"("Menu"=fg_typedef."Get") -> ("Output"=w120:T7)  [unwired: 1 in]
    n167 = feedback #8() -> (w102:T9)
    n168 = feedback-in #8(w102) -> ()
    n169 = Bundle By Name(cluster=w120, "Main mSPI"=w123) -> (w119:T7)
    n170 = call <vilib>:"WPI_MotorControlSetOutput.vi"("Output"=w93, "MotorControlDevRef"=w102) -> ()  [unwired: 7 in, 3 out]
    n171 = feedback #9() -> (w101:T9)
    n172 = feedback-in #9(w101) -> ()
    n173 = call "performance fg.vi"("Input"=w119, "Menu"=fg_typedef."Set") -> ()  [unwired: 1 out]
    n174 = call <vilib>:"WPI_MotorControlSetOutput.vi"("Output"=w96, "MotorControlDevRef"=w101) -> ()  [unwired: 7 in, 3 out]
  }
  n175 = Merge Errors("error in", w1, w10, w9, w8, w7, w6, w5, w4, w3) -> (→"error out":errorcluster)
